vi "RT-LTSM-Layer.vi"(1 "Input Array":dbl[](array[numeric]), 2 "Weights (4x4x1000x15)":dbl[][][][](array[numeric]), 3 "Layer Size":i32=15) -> (0 "Output Array":dbl[](array[numeric]))   [LabVIEW 2020]
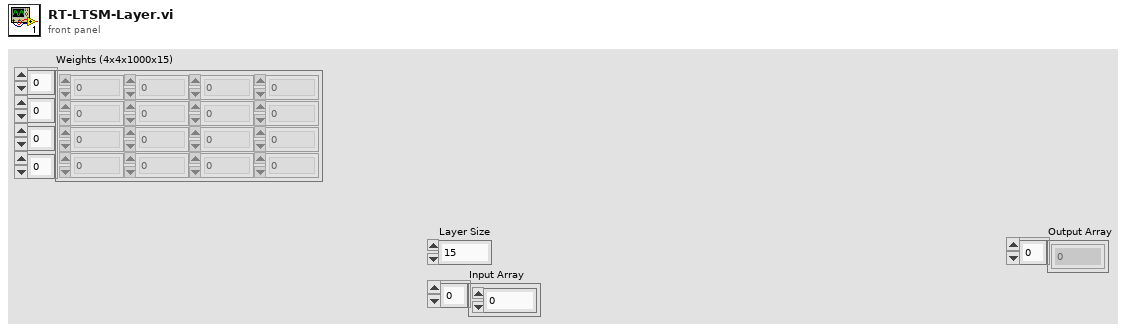
[diagram p1: front panel]
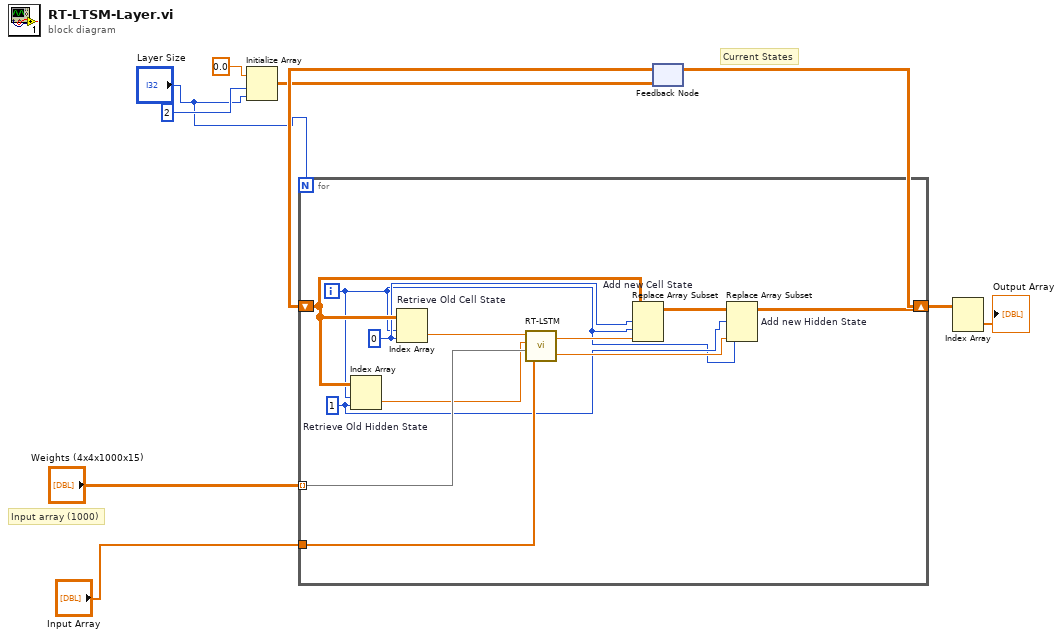
[diagram p0: block diagram]
diagram:
  # "Current States"
  # "Input array (1000)"
  n1 = Initialize Array(0.0, 2 ("dimension size"), "Layer Size") -> (w6:dbl[][])
  n2 = feedback #1(w6) -> (w7:dbl[][])
  n3 = for {
    N: "Layer Size" -> [_]
    shift-right: [w16] -> w5
    shift-left: w7 -> [w15]
    tunnel: "Input Array" -> [w21]
    tunnel: "Weights (4x4x1000x15)" -> [w20] mode=indexing
    i -> [w10]
    w11 = 1 ("disabled index (col)")
    w12 = 0 ("disabled index (col)")
    n4 = Index Array "Retrieve Old Hidden State"(array=w15, index (row)=w10, index (col)=w11) -> (element=w13:dbl)
    n5 = Index Array "Retrieve Old Cell State"(array=w15, index (row)=w10, index (col)=w12) -> (element=w14:dbl)
    n6 = call "RT-LSTM.vi"("Inputs"=w21, "Weights"=w20, "Previous Hidden State"=w13, "Previous Cell State"=w14) -> ("Hidden State"=w17:dbl, "Cell State"=w18:dbl)
    n7 = Replace Array Subset "Add new Cell State"(array=w15, new element=w18, index (row)=w12, index (col)=w10) -> (w19:dbl[][])
    n8 = Replace Array Subset "Add new Hidden State"(array=w19, new element=w17, index (row)=w11, index (col)=w10) -> (w16:dbl[][])
  }
  n9 = feedback-in #1(w5) -> ()
  n10 = Index Array(array=w5) -> (element=→"Output Array":dbl[])  [unwired: 2 in]
